vi "RobotDriveOpen6MotorWithTalonSRX.vi"(0 "Left Motor 1":u8=255, 1 "Left Motor 2":u8=255, 2 "Left Motor 3":u8=255, 3 "Right Motor 1":u8=255, 4 "Right Motor 2":u8=255, 5 "Right Motor 3":u8=255, 7 "error in (no error)":errorcluster, 8 "Left Motor 1 Inverted":bool, 9 "Right Motor 1 Inverted":bool, 10 "Left Motor 2 Inverted":bool, 11 "Right Motor 2 Inverted":bool, 12 "Left Motor 3 Inverted":bool, 13 "Right Motor 3 Inverted":bool, 14 "Control Mode":T1, 15 "Master Device Number":u8) -> (20 "RobotDriveDevRef":T2={"DevStatus"={"status"=FALSE, "code"=0, "source"=""}, "Motors[]"=[], "Square Inputs"=FALSE, "Max Output"=1.0}, 27 "error out":errorcluster)   [LabVIEW 2016]
doc: "Opens a reference to the robot drive for a two-, four-, or six-motor robot using Talon SR motor controllers connected via CAN bus.\n\nFor 2-motor drive, connect Left Motor 1 and Right Motor 1.\nFor 4-motor drive, connect Left Motor 2 and Right Motor 2 in addition to the 2-motor drive connections.\nFor 6-motor drive, connect Left Motor 3 and Right Motor 3 in addition to the 4-motor drive connections.\n\nInversions are optional and are set to false if disconnected.\n\nThis software is licensed. Open the labview\\readme\\WPI Robotics Library Open Source License.txt file for more information."
uses:
  <vilib>/Rock Robotics/WPI/RobotDrive/WPI_RobotDriveDevRef.ctl
  <vilib>/Rock Robotics/WPI/MotorControl/WPI_MotorControlDeviceRef.ctl
  <vilib>/Rock Robotics/WPI/MotorControl/WPI_MotorControlType.ctl
  <vilib>/Rock Robotics/SystemInterfaces/DIO/FPGA_DIOPWMChannel.ctl
  <vilib>/Rock Robotics/WPI/PWM/WPI_PWMDeadband.ctl
  <vilib>/Rock Robotics/WPI/ThirdParty/CanMotor/TalonSRX/WPI_CANTalonSRX_APIControlMode.ctl
  <vilib>/Rock Robotics/WPI/SafetyOutput/WPI_SafetyOutputConfigMenu.ctl
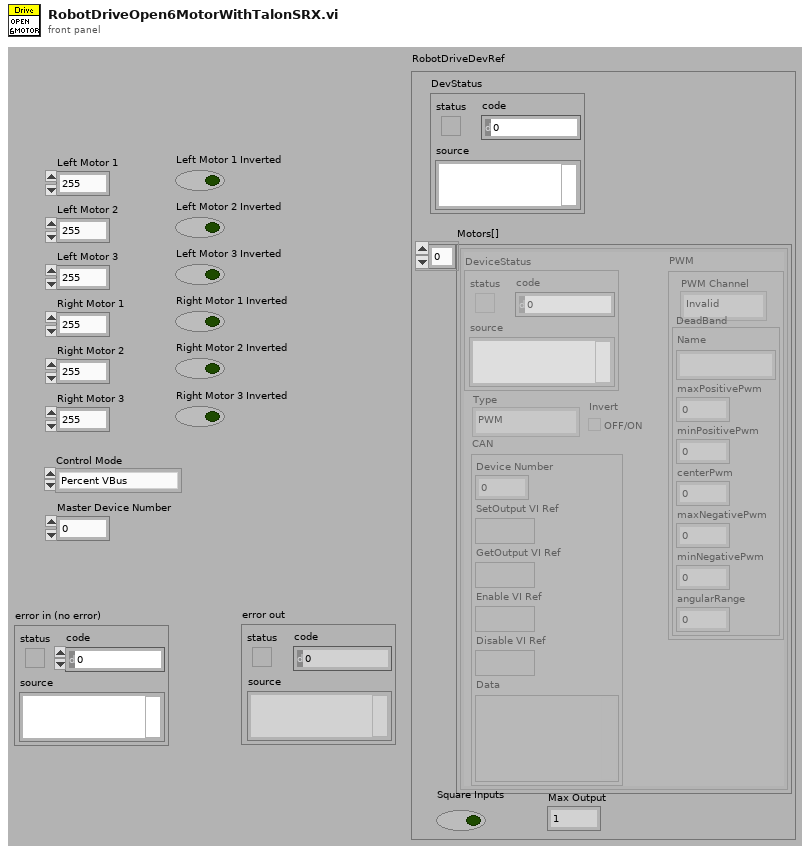
[diagram p1: front panel]
types:
  T1 = typedef "WPI_CANTalonSRX_APIControlMode.ctl" = enum8{"Percent VBus", "Speed", "Position", "Slave", "Unchanged / Invalid", "Voltage Compensation", "Current", "Motion Profile", "Motion Magic"}
  T2 = typedef "WPI_RobotDriveDevRef.ctl" = cluster{"DevStatus":errorcluster, "Motors[]":T3[], "Square Inputs":bool, "Max Output":dbl}
  T3 = typedef "WPI_MotorControlDeviceRef.ctl" = cluster{"DeviceStatus":errorcluster, "Type":T4, "PWM":cluster{"PWM Channel":T5, "DeadBand":T6}, "CAN":cluster{"Device Number":u8, "SetOutput VI Ref":variant, "GetOutput VI Ref":variant, "Enable VI Ref":variant, "Disable VI Ref":variant, "Data":variant}, "Invert":bool}
  T4 = typedef "WPI_MotorControlType.ctl" = enum16{"PWM", "CAN"}
  T5 = typedef "FPGA_DIOPWMChannel.ctl" = enum8{"PWM 0", "PWM 1", "PWM 2", "PWM 3", "PWM 4", "PWM 5", "PWM 6", "PWM 7", "PWM 8", "PWM 9", "PWM MXP 0", "PWM MXP 1", "PWM MXP 2", "PWM MXP 3", "PWM MXP 4", "PWM MXP 5", "PWM MXP 6", "PWM MXP 7", "PWM MXP 8", "PWM MXP 9", "Invalid"}
  T6 = typedef "WPI_PWMDeadband.ctl" = cluster{"Name":string, "maxPositivePwm":i32, "minPositivePwm":i32, "centerPwm":i32, "maxNegativePwm":i32, "minNegativePwm":i32, "angularRange":u16}
  T7 = typedef "WPI_SafetyOutputConfigMenu.ctl" = enum16{"Enable", "Disable"}
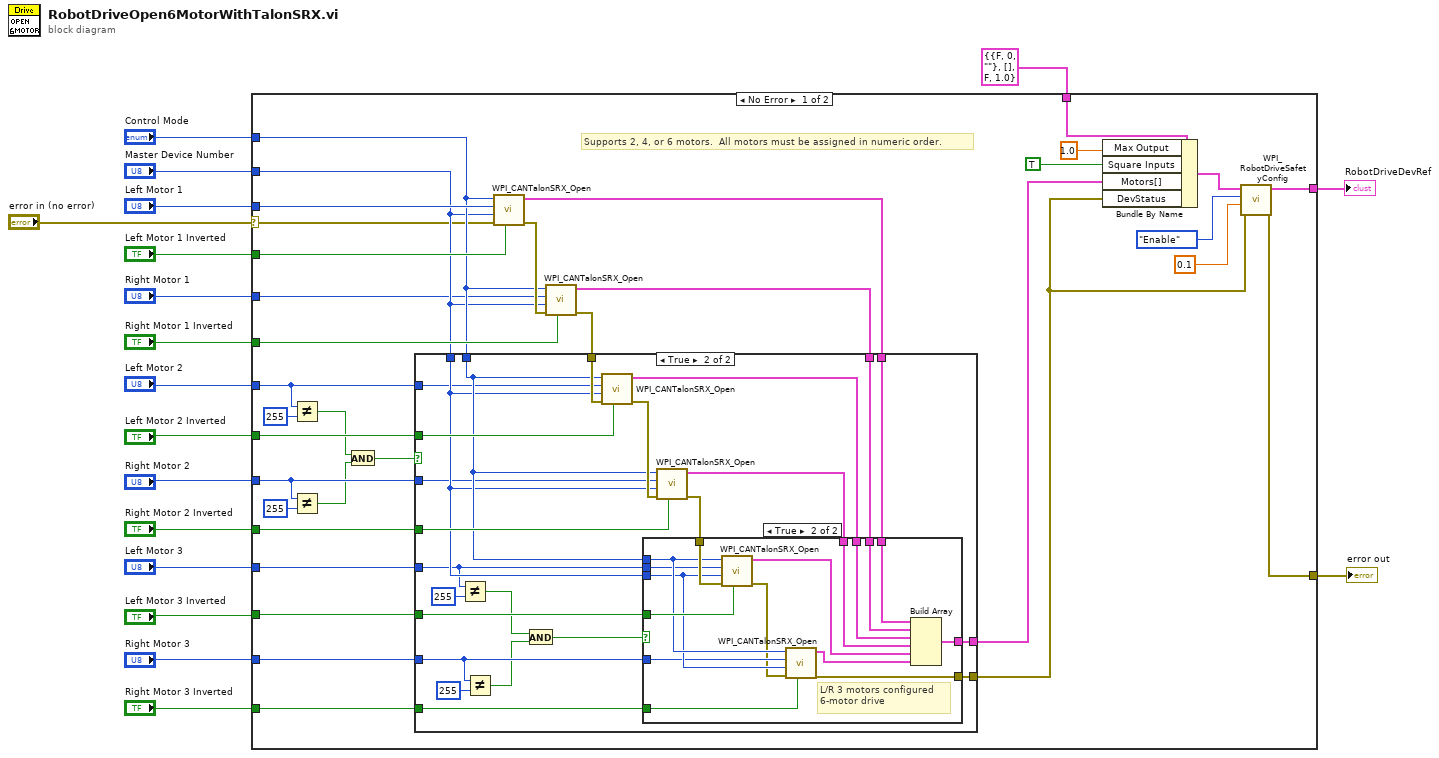
[diagram p0: block diagram]
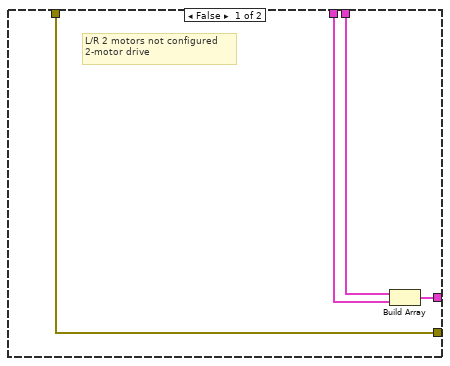
[diagram p2: hidden frame]
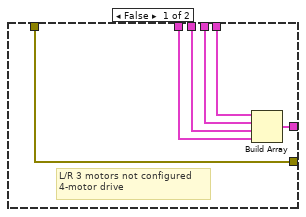
[diagram p3: hidden frame]
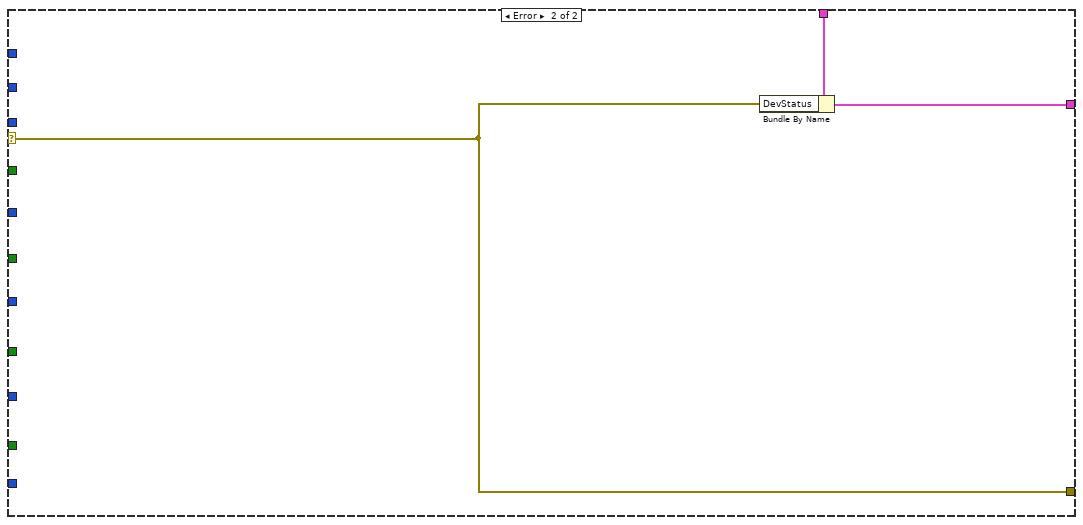
[diagram p4: hidden frame]
diagram:
  n1 = case shown="No Error" "error in (no error)" {
    selector: "error in (no error)" -> [w29 w103]
    tunnel: [w41 w104] -> w18
    tunnel: T2 {"DevStatus"={"status"=FALSE, "code"=0, "source"=""}, "Motors[]"=[], "Square Inputs"=FALSE, "Max Output"=1.0} ("RobotDriveDevRef") -> [w52 w105]
    tunnel: "Left Motor 1 Inverted" -> [w48 _]
    tunnel: "Right Motor 1 Inverted" -> [w47 _]
    tunnel: "Right Motor 2 Inverted" -> [w45 _]
    tunnel: "Left Motor 2 Inverted" -> [w46 _]
    tunnel: [w42 w103] -> w11
    tunnel: "Left Motor 3 Inverted" -> [w38 _]
    tunnel: "Right Motor 3 Inverted" -> [w37 _]
    tunnel: "Left Motor 1" -> [w35 _]
    tunnel: "Control Mode" -> [w34 _]
    tunnel: "Master Device Number" -> [w33 _]
    tunnel: "Right Motor 1" -> [w32 _]
    tunnel: "Left Motor 2" -> [w28 _]
    tunnel: "Right Motor 2" -> [w25 _]
    tunnel: "Left Motor 3" -> [w31 _]
    tunnel: "Right Motor 3" -> [w30 _]
    frame No Error {
      # "Supports 2, 4, or 6 motors.  All motors must be assigned in numeric order."
      n2 = Not Equal?(x=w28, y=u8 255) -> (x != y?=w24:bool)
      n3 = Not Equal?(x=w25, y=u8 255) -> (x != y?=w23:bool)
      n4 = And(x=w24, y=w23) -> (x .and. y?=w22:bool)
      n5 = call <vilib>:"WPI_CANTalonSRX_Open.vi"("Invert"=w48, "error in"=w29, "Master Device Number"=w33, "Device Number"=w35, "Control Mode"=w34) -> ("error out"=w49:errorcluster, "CAN Talon SRX Ref"=w20:T3)  [unwired: 5 in]
      n6 = call <vilib>:"WPI_CANTalonSRX_Open.vi"("Invert"=w47, "error in"=w49, "Master Device Number"=w33, "Device Number"=w32, "Control Mode"=w34) -> ("error out"=w50:errorcluster, "CAN Talon SRX Ref"=w19:T3)  [unwired: 5 in]
      n7 = case shown="True" w22 {
        tunnel: w50 -> [w56 w79]
        tunnel: w46 -> [_ w78]
        tunnel: w45 -> [_ w77]
        tunnel: w38 -> [_ w75]
        tunnel: w37 -> [_ w74]
        tunnel: [w56 w73] -> w36
        tunnel: w34 -> [_ w72]
        tunnel: w33 -> [_ w71]
        tunnel: w31 -> [_ w65]
        tunnel: w30 -> [_ w66]
        tunnel: w28 -> [_ w70]
        tunnel: w25 -> [_ w69]
        tunnel: [w55 w61] -> w21
        tunnel: w20 -> [w54 w60]
        tunnel: w19 -> [w53 w59]
        frame False {
          # "L/R 2 motors not configured\n2-motor drive"
          n8 = Build Array(w54, w53) -> (w55:T3[])
        }
        frame True {
          n9 = Not Equal?(x=w65, y=u8 255) -> (x != y?=w63:bool)
          n10 = Not Equal?(x=w66, y=u8 255) -> (x != y?=w62:bool)
          n11 = And(x=w63, y=w62) -> (x .and. y?=w64:bool)
          n12 = call <vilib>:"WPI_CANTalonSRX_Open.vi"("Invert"=w78, "error in"=w79, "Master Device Number"=w71, "Device Number"=w70, "Control Mode"=w72) -> ("error out"=w80:errorcluster, "CAN Talon SRX Ref"=w58:T3)  [unwired: 5 in]
          n13 = call <vilib>:"WPI_CANTalonSRX_Open.vi"("Invert"=w77, "error in"=w80, "Master Device Number"=w71, "Device Number"=w69, "Control Mode"=w72) -> ("error out"=w76:errorcluster, "CAN Talon SRX Ref"=w57:T3)  [unwired: 5 in]
          n14 = case shown="True" w64 {
            tunnel: w76 -> [w86 w102]
            tunnel: w75 -> [_ w101]
            tunnel: w74 -> [_ w100]
            tunnel: [w86 w99] -> w73
            tunnel: w72 -> [_ w98]
            tunnel: w71 -> [_ w97]
            tunnel: w65 -> [_ w96]
            tunnel: w66 -> [_ w95]
            tunnel: [w85 w93] -> w61
            tunnel: w60 -> [w84 w92]
            tunnel: w59 -> [w83 w91]
            tunnel: w58 -> [w82 w90]
            tunnel: w57 -> [w81 w89]
            frame False {
              # "L/R 3 motors not configured\n4-motor drive"
              n15 = Build Array(w84, w83, w82, w81) -> (w85:T3[])
            }
            frame True {
              # "L/R 3 motors configured\n6-motor drive"
              n16 = call <vilib>:"WPI_CANTalonSRX_Open.vi"("Invert"=w101, "error in"=w102, "Master Device Number"=w97, "Device Number"=w96, "Control Mode"=w98) -> ("error out"=w94:errorcluster, "CAN Talon SRX Ref"=w88:T3)  [unwired: 5 in]
              n17 = call <vilib>:"WPI_CANTalonSRX_Open.vi"("Invert"=w100, "error in"=w94, "Master Device Number"=w97, "Device Number"=w95, "Control Mode"=w98) -> ("error out"=w99:errorcluster, "CAN Talon SRX Ref"=w87:T3)  [unwired: 5 in]
              n18 = Build Array(w92, w91, w90, w89, w88, w87) -> (w93:T3[])
            }
          }
        }
      }
      n19 = Bundle By Name(cluster=w52, "Max Output"=1.0, "Square Inputs"=TRUE ("DestroyPWM?"), "Motors[]"=w21, "DevStatus"=w36) -> (w43:T2)
      n20 = call <vilib>:"WPI_RobotDriveSafetyConfig.vi"("error in (no error)"=w36, "timeout (s)"=0.1, "mode"=WPI_SafetyOutputConfigMenu."Enable", "RobotDriveDevRef"=w43) -> ("error out"=w42:errorcluster, "RobotDriveDevRef"=w41:T2)  [unwired: 6 out]
    }
    frame Error {
      n21 = Bundle By Name(cluster=w105, "DevStatus"=w103) -> (w104:T2)
    }
  }
  "RobotDriveDevRef" <- w18
  "error out" <- w11
